vi "Configure Resistance.vi"(6 "Enable Offset Compensation (F: Disable)":bool, 7 "Enable Power Limit (F: Disable)":bool, 8 "error in (no error)":errorcluster, 9 "Resistance Integration Time (10: 10)":dbl(ring)=10.0 items=["0.02"=0.02, "0.2"=0.2, "1"=1.0, "10"=10.0, "100"=100.0], 10 "Resistance Type (0: Resistance 2-wire)":i32(ring) items=["Resistance 2-wire", "Resistance 4-wire"], 11 "VISA resource name":refnum<visa-resource-name>) -> (0 "error out":errorcluster, 3 "VISA resource name out":refnum<visa-resource-name>)   [LabVIEW 2013, in "Agilent 3446X Series.lvlib"]
doc: "Configures the settings for resistance measurements.\n\n<b>Note(s) : </b>\nFor EDU34450A model Offset Compensation only supported."
uses:
  <instrlib>/Agilent 3446X Series/Agilent 3446X Series.lvlib
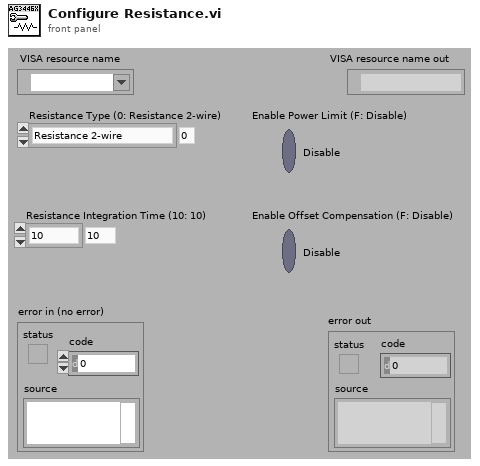
[diagram p1: front panel]
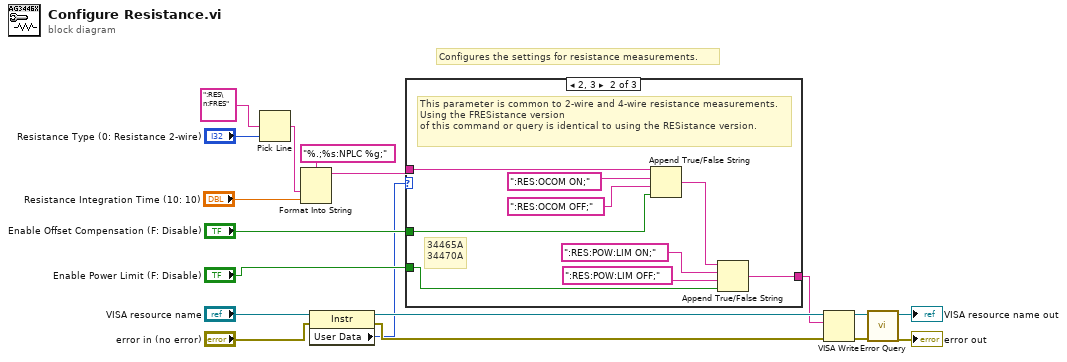
[diagram p0: block diagram]
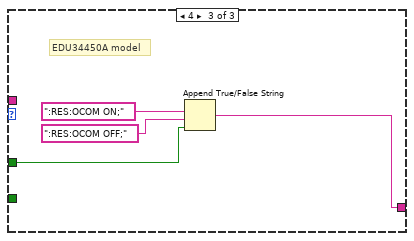
[diagram p3: hidden frame]
diagram:
  # "Configures the settings for resistance measurements."
  n1 = Pick Line(multi-line string=":RES\n:FRES", line index="Resistance Type (0: Resistance 2-wire)") -> (output string=w3:string)  [unwired: 1 out]
  n2 = Format Into String(format string="%.;%s:NPLC %g;", w3, "Resistance Integration Time (10: 10)") -> (resulting string=w1:string)  [unwired: 2 in, 1 out]
  n3 = property class="Instr"(reference="VISA resource name", error in="error in (no error)") -> (reference out=w9:refnum<visa-resource-name>, error out=w8:errorcluster, "User Data"=w6:u32)
  n4 = case shown="2, 3" w6 {
    tunnel: [w19 w21 w29] -> w5
    tunnel: "Enable Offset Compensation (F: Disable)" -> [_ w23 w30]
    tunnel: "Enable Power Limit (F: Disable)" -> [_ w22 _]
    tunnel: w1 -> [w19 w20 _]
    frame 0, 1, Default {
      # "34460A\n34461A"
    }
    frame 2, 3 {
      # "34465A\n34470A"
      # "This parameter is common to 2-wire and 4-wire resistance measurements. Using the FRESistance version\nof this command or query is identical to using the RESistance version."
      n5 = Append True/False String(1:w23, 2:":RES:OCOM OFF;" ("true string"), 3:":RES:OCOM ON;" ("true string"), 4:w20) -> (0:w28:string)
      n6 = Append True/False String(1:w22, 2:":RES:POW:LIM OFF;" ("true string"), 3:":RES:POW:LIM ON;" ("true string"), 4:w28) -> (0:w21:string)
    }
    frame 4 {
      # "EDU34450A model"
      n7 = Append True/False String(1:w30, 2:":RES:OCOM OFF;" ("true string"), 3:":RES:OCOM ON;" ("true string")) -> (0:w29:string)  [unwired: 1 in]
    }
  }
  n8 = VISA Write(VISA resource name=w9, write buffer=w5, error in (no error)=w8) -> (VISA resource name out=w16:refnum<visa-resource-name>, error out=w15:errorcluster)  [unwired: 1 out]
  n9 = call <instrlib>:"Error Query.vi"("error in (no error)"=w15, "VISA resource name"=w16) -> ("error out"=→"error out":errorcluster, "VISA resource name out"=→"VISA resource name out":refnum<visa-resource-name>)  [unwired: 8 out]
